vi "Configure Calib Linear (Com).vi"(0 "VISA resource name":refnum<visa-resource-name>, 5 "Channel (001)":string="001", 7 "Mode (0: Off)":u16(ring) items=["Off", "Apporoximation", "Bias"], 9 "Linearizer Input/Output":cluster{"Input":i32, "Output":i32}[](array[cluster]) {"Output" min=-999999 max=999999; "Input" min=-999999 max=999999}, 11 "error in (no error)":errorcluster) -> (4 "VISA resource name out":refnum<visa-resource-name>, 6 "Channel":string, 15 "error out":errorcluster)   [LabVIEW 2020, in "Yokogawa GX Series.lvlib"]
doc: "Sets the calibration correction(Linearizer Approximation and Linearizer Bias) for communication channels.\n\nCommand: SCalibUseCom, SCalibCom"
uses:
  <instrlib>/Yokogawa GX Series/Yokogawa GX Series.lvlib
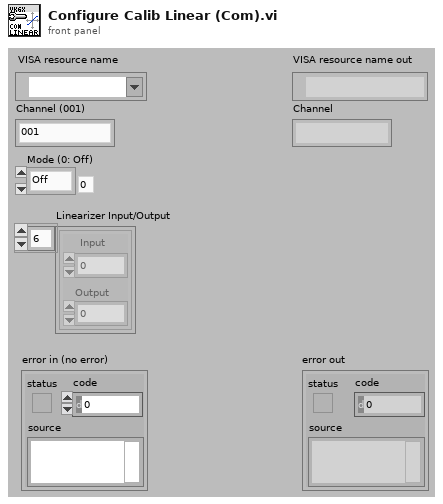
[diagram p1: front panel]
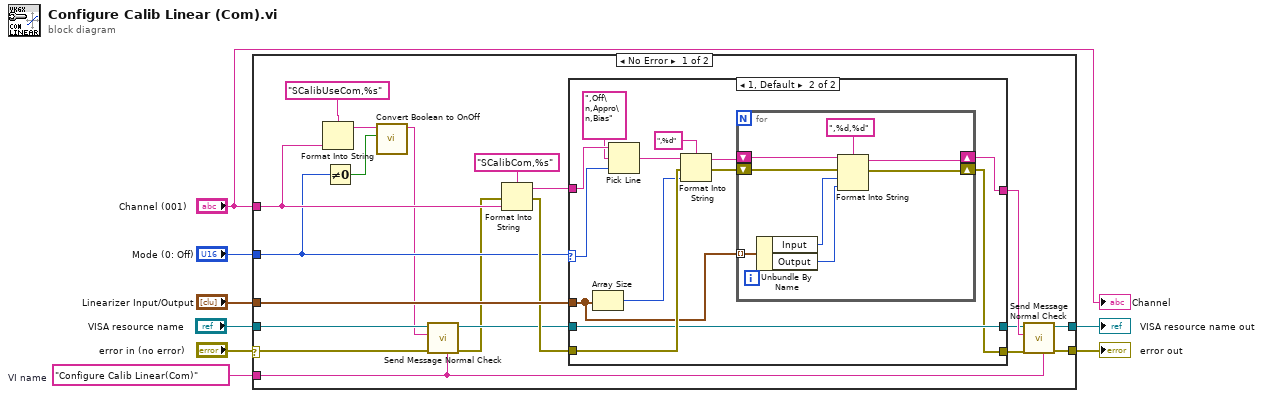
[diagram p0: block diagram]
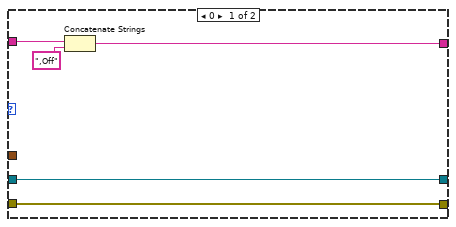
[diagram p2: hidden frame]
diagram:
  w8 = "Configure Calib Linear(Com)"  # VI name
  n1 = case shown="No Error" "error in (no error)" {
    selector: "error in (no error)" -> [w11 w55]
    tunnel: w8 -> [w9 _]
    tunnel: [w28 w56] -> w7
    tunnel: [w27 w55] -> w6
    tunnel: "VISA resource name" -> [w13 w56]
    tunnel: "Mode (0: Off)" -> [w16 _]
    tunnel: "Linearizer Input/Output" -> [w25 _]
    tunnel: "Channel (001)" -> [w17 _]
    frame No Error {
      n2 = Format Into String(format string="SCalibUseCom,%s", w17) -> (resulting string=w20:string)  [unwired: 2 in, 1 out]
      n3 = Not Equal To 0?(x=w16) -> (x != 0?=w15:bool)
      n4 = call <instrlib>:"Convert Boolean to OnOff.vi"("On/Off"=w15, "Initial String (\"\")"=w20) -> ("Resulting String"=w10:string)  [unwired: 9 in]
      n5 = call <instrlib>:"Send Message Normal Check.vi"("Source (\"\")"=w9, "error in (no error)"=w11, "Send Message (\"\")"=w10, "VISA resource name"=w13) -> ("error out"=w12:errorcluster, "VISA resource name out"=w14:refnum<visa-resource-name>)  [unwired: 2 in, 4 out]
      n6 = Format Into String(format string="SCalibCom,%s", error in=w12, w17) -> (resulting string=w26:string, error out=w24:errorcluster)  [unwired: 1 in]
      n7 = case shown="1, Default" w16 {
        selector: w16 -> [_ w46]
        tunnel: w26 -> [w33 w45]
        tunnel: [w31 w37] -> w23
        tunnel: w25 -> [_ w39]
        tunnel: w24 -> [w29 w41]
        tunnel: w14 -> [w30 w36]
        tunnel: [w30 w36] -> w22
        tunnel: [w29 w35] -> w21
        frame 0 {
          n8 = Concatenate Strings(w33, ",Off") -> (w31:string)
        }
        frame 1, Default {
          n9 = Array Size(array=w39) -> (size(s)=w34:i32)
          n10 = Pick Line(string ("")=w45, multi-line string=",Off\n,Appro\n,Bias", line index=w46) -> (output string=w42:string)
          n11 = Format Into String(format string=",%d", initial string=w42, error in=w41, w34) -> (resulting string=w40:string, error out=w38:errorcluster)
          n12 = for {
            tunnel: w39 -> [w52] mode=indexing
            shift-right: [w48] -> w37
            shift-left: w40 -> [w54]
            shift-right: [w49] -> w35
            shift-left: w38 -> [w53]
            n13 = Unbundle By Name(w52) -> ("Input"=w51:i32, "Output"=w50:i32)
            n14 = Format Into String(format string=",%d,%d", initial string=w54, error in=w53, w51, w50) -> (resulting string=w48:string, error out=w49:errorcluster)
          }
        }
      }
      n15 = call <instrlib>:"Send Message Normal Check.vi"("Source (\"\")"=w9, "error in (no error)"=w21, "Send Message (\"\")"=w23, "VISA resource name"=w22) -> ("error out"=w27:errorcluster, "VISA resource name out"=w28:refnum<visa-resource-name>)  [unwired: 2 in, 4 out]
    }
    frame Error {
    }
  }
  "error out" <- w6
  "VISA resource name out" <- w7
  "Channel" <- "Channel (001)"
